vi "CLSUIP_ResizeBDWin.vi"(7 "VIRetooler in":refnum<class "VIRetooler.lvclass">, 8 "error in (no error)":errorcluster, 11 "VI Refnum":refnum<vi>) -> (0 "error out":errorcluster, 3 "VI Refnum out":refnum<vi>)   [LabVIEW 2021, in "MemberVICreation.lvlib" / "VIRetooler.lvclass"]
uses:
  <resource>/Framework/Providers/LVClassLibrary/NewAccessors/VIRetooler/VIRetooler.lvclass
  <resource>/Framework/Providers/LVClassLibrary/NewAccessors/MemberVICreation.lvlib
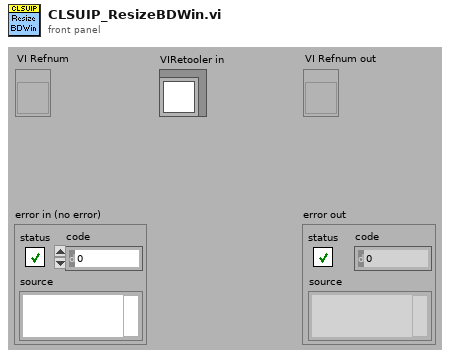
[diagram p1: front panel]
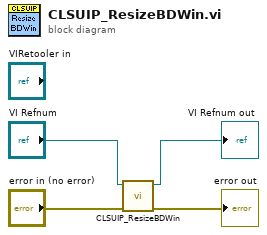
[diagram p0: block diagram]
diagram:
  n1 = call <resource>:"CLSUIP_ResizeBDWin.vi"("error in (no error)"="error in (no error)", "VI Refnum"="VI Refnum") -> ("error out"=→"error out":errorcluster, "VI Refnum out"=→"VI Refnum out":refnum<vi>)  [unwired: 8 out]
